vi "Driver.vi"(11 "JoystickDevRef in":T1) -> (2 "Output":cluster{"Left":dbl, "Right":dbl}, 3 "JoystickDevRef out":T1)   [LabVIEW 2016]
uses:
  <vilib>/Rock Robotics/WPI/Joystick/WPI_JoystickDevRef.ctl
  <vilib>/Rock Robotics/WPI/Joystick/WPI_JoystickDeviceEnum.ctl
  <vilib>/Rock Robotics/Network Tables/NT Write Numeric Array.vi
  <vilib>/Rock Robotics/Network Tables/NT Write Boolean Array.vi
panel:
  out "Select  PlaceHolder":bool
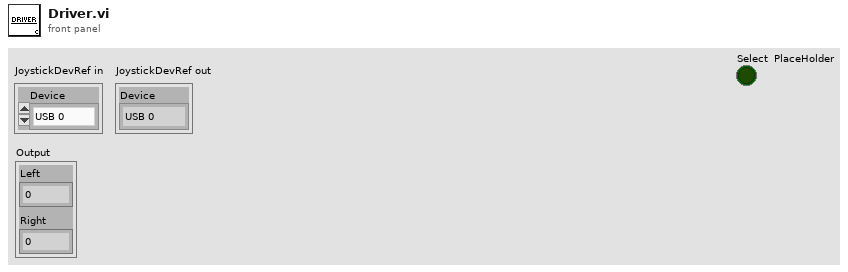
[diagram p1: front panel]
types:
  T1 = typedef "WPI_JoystickDevRef.ctl" = cluster{"Device":T2}
  T2 = typedef "WPI_JoystickDeviceEnum.ctl" = enum16{"USB 0", "USB 1", "USB 2", "USB 3", "USB 4", "USB 5"}
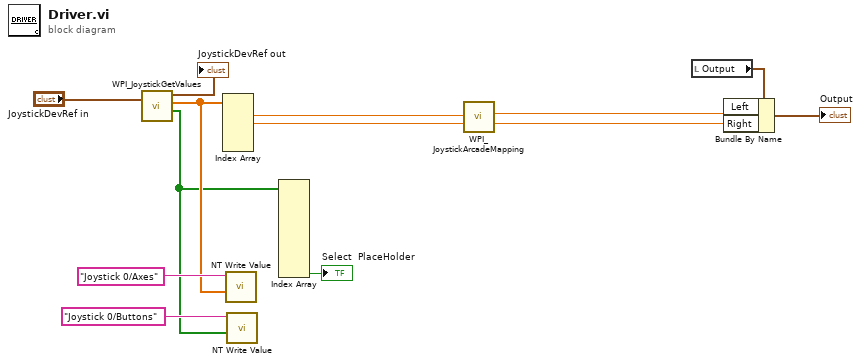
[diagram p0: block diagram]
diagram:
  n1 = call <vilib>:"WPI_JoystickGetValues.vi"("JoystickDevRef"="JoystickDevRef in") -> ("Buttons"=w6:bool[], "Axes"=w11:dbl[], "JoystickDevRef"=→"JoystickDevRef out":T1)  [unwired: 6 in, 2 out]
  n2 = Index Array(array=w11) -> (element #1=w8:dbl, element #2=w7:dbl)  [unwired: 5 in, 3 out]
  n3 = call-poly <vilib>:"NT Write Value.vi"("Numeric Array"=w11, "Name"="Joystick 0/Axes") -> ()  [unwired: 9 in, 1 out]
  n4 = call-poly <vilib>:"NT Write Value.vi"("Boolean Array"=w6, "Name"="Joystick 0/Buttons") -> ()  [unwired: 9 in, 1 out]
  n5 = Index Array(array=w6) -> (element #10=→"Select  PlaceHolder":bool)  [unwired: 10 in, 9 out]
  n6 = call <vilib>:"WPI_JoystickArcadeMapping.vi"("Y axis value"=w7, "X axis value"=w8) -> ("Right Motor Value"=w1:dbl, "Left Motor Value"=w4:dbl)  [unwired: 8 in]
  n7 = local read "Output"() -> (w2:cluster{"Left":dbl, "Right":dbl})
  n8 = Bundle By Name(cluster=w2, "Left"=w4, "Right"=w1) -> (→"Output":cluster{"Left":dbl, "Right":dbl})
